vi "Check temperature warnings.vi"(6 "Inner coil limit [K]":dbl=9.0, 8 "Outer coil limit [K]":dbl=9.0, 9 "1st Cryocooler limit [K]":dbl=50.0, 10 "2nd cryocooler limit [K]":dbl=8.0, 11 "LSC218 sensors":T1 {"Time stamp" format="%<%H:%M:%S%2u\n%Y/%m/%d>T"}) -> (1 "Time stamp":dbl format="%<%H:%M:%S%3u\n%Y/%m/%d>T", 2 "Coil Overheat":bool, 3 "Crocooler overheat":bool)   [LabVIEW 2022 SP3, in "Magnet module.lvlib"]
doc: "Evaluates overheat warnings.\nCompares actual temperatures from sensors with constants from configuration file."
uses:
  Magnet module.lvlib
  ctl/Cryostat temperature sensors.ctl
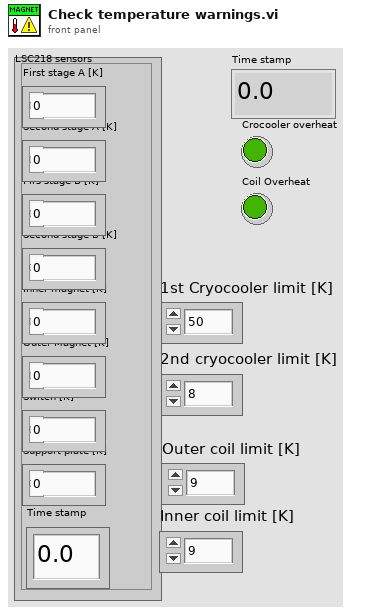
[diagram p1: front panel]
types:
  T1 = typedef "Magnet module.lvlib/Cryostat temperature sensors.ctl" = cluster{"First stage A [K]":dbl, "Second stage A [K]":dbl, "Firs stage B [K]":dbl, "Second stage B [K]":dbl, "Inner magnet [K]":dbl, "Outer Magnet [K]":dbl, "Switch [K]":dbl, "Support plate [K]":dbl, "Time stamp":dbl}
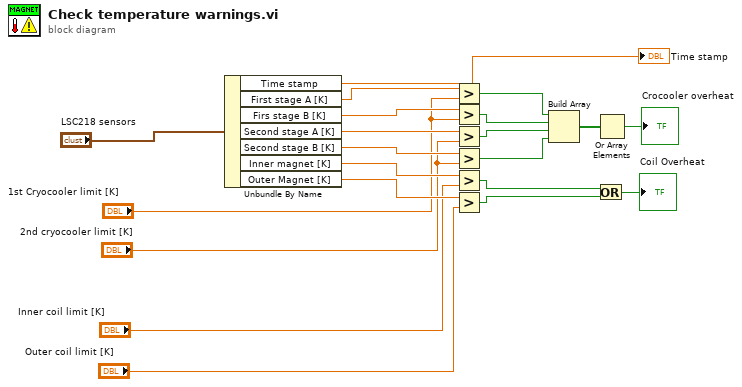
[diagram p0: block diagram]
diagram:
  n1 = Unbundle By Name("LSC218 sensors") -> ("Time stamp"=→"Time stamp":dbl, "First stage A [K]"=w5:dbl, "Firs stage B [K]"=w8:dbl, "Second stage A [K]"=w9:dbl, "Second stage B [K]"=w10:dbl, "Inner magnet [K]"=w11:dbl, "Outer Magnet [K]"=w12:dbl)
  n2 = Greater?(x=w5, y="1st Cryocooler limit [K]") -> (0:w13:bool)
  n3 = Greater?(x=w8, y="1st Cryocooler limit [K]") -> (0:w14:bool)
  n4 = Greater?(x=w9, y="2nd cryocooler limit [K]") -> (0:w15:bool)
  n5 = Greater?(x=w10, y="2nd cryocooler limit [K]") -> (0:w16:bool)
  n6 = Greater?(x=w11, y="Inner coil limit [K]") -> (0:w18:bool)
  n7 = Greater?(x=w12, y="Outer coil limit [K]") -> (0:w19:bool)
  n8 = Build Array(w13, w14, w15, w16) -> (w17:bool[])
  n9 = Or(x=w18, y=w19) -> (x .or. y?=→"Coil Overheat":bool)
  n10 = Or Array Elements(Boolean array=w17) -> (logical OR=→"Crocooler overheat":bool)
